vi "FTW-Reflection-TypeDescriptorToDefaultData.vi"(7 "Type Descriptor":i16[](array[numeric]) format="%04x") -> (8 "Variant Type Default Value":variant)   [LabVIEW 2014]
panel:
  # "Inputs"
  # "Outputs"
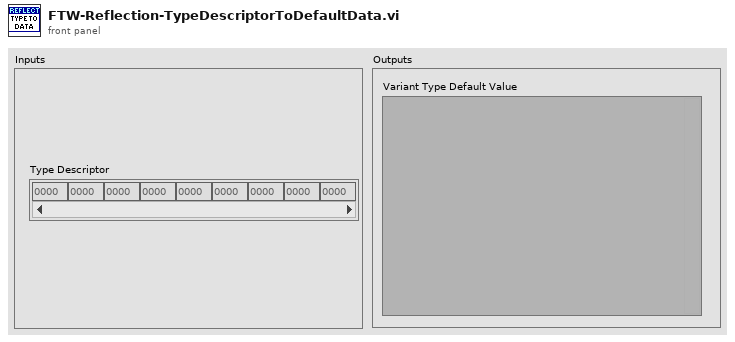
[diagram p1: front panel]
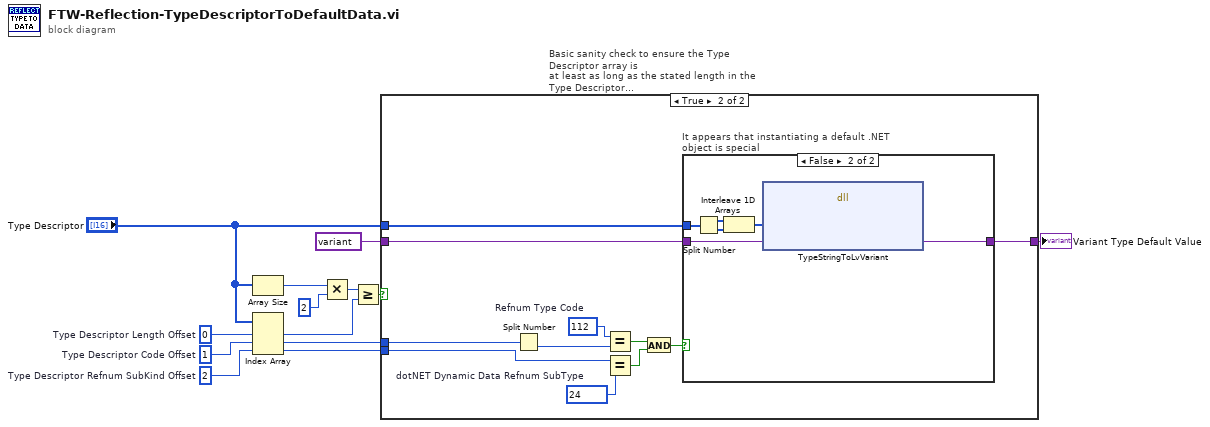
[diagram p0: block diagram]
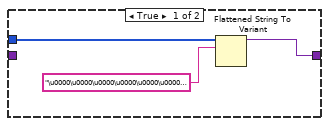
[diagram p3: hidden frame]
diagram:
  w1 = 2  # Type Descriptor Refnum SubKind Offset
  w4 = 1  # Type Descriptor Code Offset
  w6 = 0  # Type Descriptor Length Offset
  n1 = Array Size(array="Type Descriptor") -> (size(s)=w9:i32)
  n2 = Index Array(array="Type Descriptor", index #1=w6, index #2=w4, index #3=w1) -> (element #1=w7:i16, element #2=w3:i16, element #3=w2:i16)
  n3 = Multiply(x=w9, y=2) -> (x*y=w8:i32)
  n4 = Greater Or Equal?(x=w8, y=w7) -> (x >= y?=w5:bool)
  n5 = case "Basic sanity check to ensure the Type Descriptor array is\nat least as long as the stated length in the Type Descriptor\nheader, since this function does not protect against overrun." shown="True" w5 {
    tunnel: variant -> [w14 w25]
    tunnel: [w14 w24] -> w12
    tunnel: "Type Descriptor" -> [_ w23]
    tunnel: w3 -> [_ w22]
    tunnel: w2 -> [_ w19]
    frame False {
    }
    frame True {
      w18 = i16 24  # dotNET Dynamic Data Refnum SubType
      w20 = u8 112  # Refnum Type Code
      n6 = Split Number(x=w22) -> (lo(x)=w21:u8)  [unwired: 1 out]
      n7 = Equal?(x=w20, y=w21) -> (x = y?=w17:bool)
      n8 = Equal?(x=w19, y=w18) -> (x = y?=w16:bool)
      n9 = And(x=w17, y=w16) -> (x .and. y?=w15:bool)
      n10 = case "It appears that instantiating a default .NET object is special" shown="False" w15 {
        tunnel: w25 -> [_ w34]
        tunnel: [w26 w30] -> w24
        tunnel: w23 -> [w28 w29]
        frame True {
          n11 = Flattened String To Variant(6:"\u0000\u0000\u0000\u0000\u0000\u0000\u0000\u0000" ("data string"), 7:w28) -> (3:w26:variant)  [unwired: 1 in, 1 out]
        }
        frame False {
          n12 = Split Number(x=w29) -> (hi(x)=w32:u8[], lo(x)=w33:u8[])
          n13 = Interleave 1D Arrays(w32, w33) -> (w31:u8[])
          n14 = dll-call lib="LabVIEW" fn="TypeStringToLvVariant"("Type Descriptor (byte array)"=w31, "Default Data"=w34) -> ("Default Data"=w30:variant)  [unwired: 5 in, 2 out]
        }
      }
    }
  }
  "Variant Type Default Value" <- w12
